vi "Add New UI.vi"(8 "error in (no error)":errorcluster, 9 "Name":string, 10 "UI Reference":refnum<vi>, 11 "SubPanel User Interface in":refnum<class "SubPanel User Interface.lvclass">) -> (0 "error out":errorcluster, 3 "SubPanel User Interface out":refnum<class "SubPanel User Interface.lvclass">)   [LabVIEW 2019, in "SubPanel User Interface.lvlib" / "SubPanel User Interface.lvclass"]
uses:
  SubPanel User Interface.lvclass
  SubPanel User Interface.lvclass/SubPanel User Interface.ctl
  UI Reference Wrapper/UI Reference Wrapper.lvclass
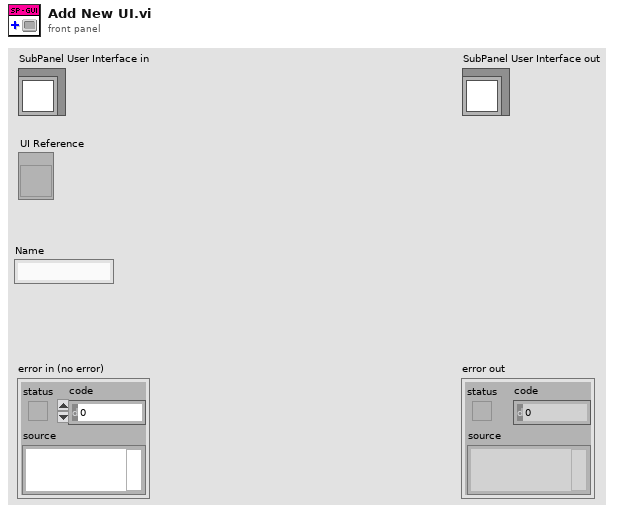
[diagram p1: front panel]
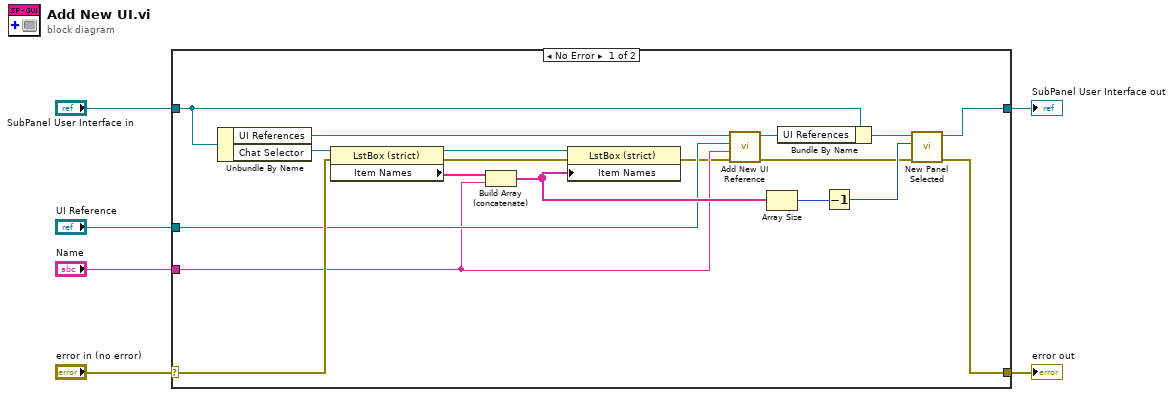
[diagram p0: block diagram]
diagram:
  n1 = case shown="No Error" "error in (no error)" {
    selector: "error in (no error)" -> [w20 w26]
    tunnel: [w17 w26] -> w5
    tunnel: [w16 w25] -> w3
    tunnel: "SubPanel User Interface in" -> [w19 w25]
    tunnel: "Name" -> [w9 _]
    tunnel: "UI Reference" -> [w10 _]
    frame No Error {
      n2 = Unbundle By Name(w19) -> ("UI References"=w12:refnum<class "UI Reference Wrapper.lvclass">, "Chat Selector"=w24:refnum<vi>)
      n3 = property class="LstBox (strict)"(reference=w24, error in=w20) -> (reference out=w23:refnum<vi>, error out=w21:errorcluster, "Item Names"=w22:string[])
      n4 = Build Array (concatenate)(w22, w9) -> (w15:string[])
      n5 = property class="LstBox (strict)"(reference=w23, error in=w21, "Item Names"=w15) -> (error out=w7:errorcluster)  [unwired: 1 out]
      n6 = call "Add New UI Reference.vi"("error in (no error)"=w7, "Name"=w9, "VI Refnum"=w10, "UI Reference Wrapper in"=w12) -> ("error out"=w8:errorcluster, "UI Reference Wrapper out"=w11:refnum<class "UI Reference Wrapper.lvclass">)  [unwired: 6 in]
      n7 = Array Size(array=w15) -> (size(s)=w14:i32)
      n8 = Bundle By Name(cluster=w19, "UI References"=w11) -> (w18:refnum<class "SubPanel User Interface.lvclass">)
      n9 = Decrement(x=w14) -> (x-1=w13:i32)
      n10 = call "New Panel Selected.vi"("error in (no error)"=w8, "Chat Window"=w13, "SubPanel User Interface in"=w18) -> ("error out"=w17:errorcluster, "SubPanel User Interface out"=w16:refnum<class "SubPanel User Interface.lvclass">)  [unwired: 7 in]
    }
    frame Error {
    }
  }
  "error out" <- w5
  "SubPanel User Interface out" <- w3
